vi "AssignToConPane.vi"(8 "error in":errorcluster, 9 "Control Refnums":refnum<vi>[](array[refnum]), 10 "Terminals":u32[](array[numeric]), 11 "ConnectorPane in":refnum<vi>) -> (0 "error out":errorcluster, 3 "ConnectorPane out":refnum<vi>)   [LabVIEW 2016]
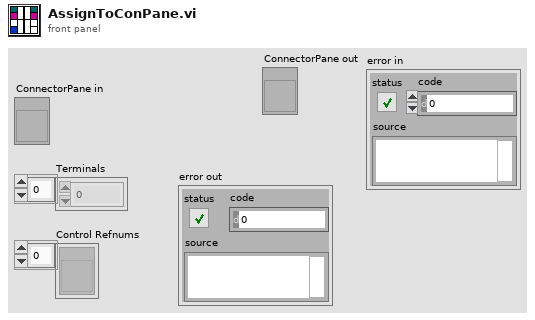
[diagram p1: front panel]
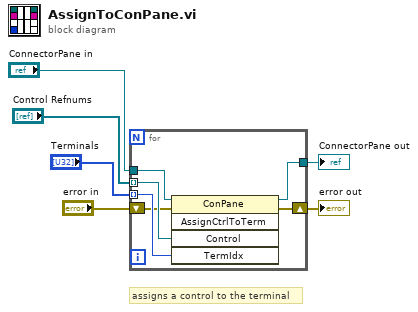
[diagram p0: block diagram]
diagram:
  # "assigns a control to the terminal"
  n1 = for {
    tunnel: "ConnectorPane in" -> [w12]
    tunnel: [w10] -> w2
    tunnel: "Control Refnums" -> [w9] mode=indexing
    tunnel: "Terminals" -> [w8] mode=indexing
    shift-right: [w11] -> w5
    shift-left: "error in" -> [w7]
    n2 = invoke class="ConPane" method="AssignCtrlToTerm"(reference=w12, error in=w7, "Control"=w9, "TermIdx"=w8) -> (reference out=w10:refnum<vi>, error out=w11:errorcluster)  [unwired: 1 in, 3 out]
  }
  "error out" <- w5
  "ConnectorPane out" <- w2
